vi "PPSU DC On.vi"(8 "Error in":errorcluster, 11 "Device information":string[](array[string])) -> (0 "Error out":errorcluster, 3 "Device information out":string[](array[string]))   [LabVIEW 2022 SP3]
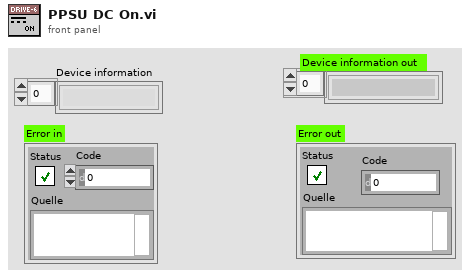
[diagram p1: front panel]
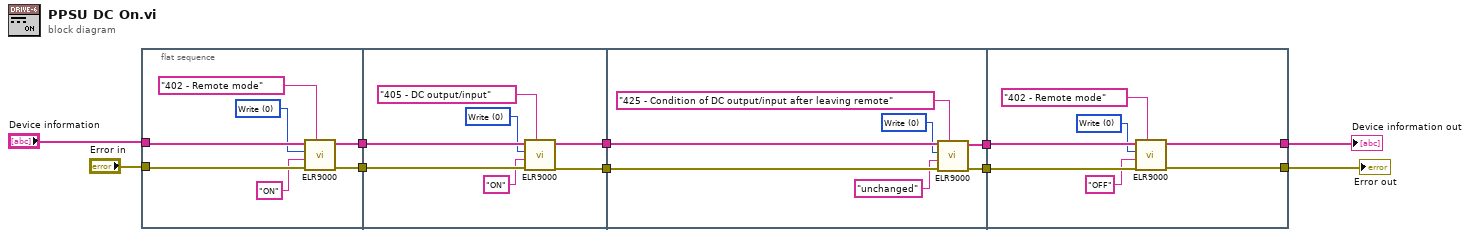
[diagram p0: block diagram]
diagram:
  n1 = flat-sequence {
    tunnel: "Error in" -> [w17]
    tunnel: "Device information" -> [w16]
    tunnel: [w12] -> w10
    tunnel: [w11] -> w9
    tunnel: w10 -> [w24]
    tunnel: w9 -> [w23]
    tunnel: [w19] -> w8
    tunnel: [w18] -> w7
    tunnel: w8 -> [w31]
    tunnel: w7 -> [w30]
    tunnel: [w26] -> w6
    tunnel: [w25] -> w5
    tunnel: w6 -> [w38]
    tunnel: w5 -> [w37]
    tunnel: [w33] -> w2
    tunnel: [w32] -> w1
    frame #0 {
      w14 = u8 0 items=["Write", "Read"] ("Access")
      n2 = call <vilib>:"ELR9000.vi"("Command list"="402 - Remote mode", "Error in"=w17, "Value"="ON", "Access"=w14, "Device information in"=w16) -> ("Error out"=w11:errorcluster, "Device information out"=w12:string[])  [unwired: 1 in, 2 out]
    }
    frame #1 {
      w21 = u8 0 items=["Write", "Read"] ("Access")
      n3 = call <vilib>:"ELR9000.vi"("Command list"="405 - DC output/input", "Error in"=w23, "Value"="ON", "Access"=w21, "Device information in"=w24) -> ("Error out"=w19:errorcluster, "Device information out"=w18:string[])  [unwired: 1 in, 2 out]
    }
    frame #2 {
      w29 = u8 0 items=["Write", "Read"] ("Access")
      n4 = call <vilib>:"ELR9000.vi"("Command list"="425 - Condition of DC output/input after leaving remote", "Error in"=w31, "Value"="unchanged", "Access"=w29, "Device information in"=w30) -> ("Error out"=w26:errorcluster, "Device information out"=w25:string[])  [unwired: 1 in, 2 out]
    }
    frame #3 {
      w35 = u8 0 items=["Write", "Read"] ("Access")
      n5 = call <vilib>:"ELR9000.vi"("Command list"="402 - Remote mode", "Error in"=w38, "Value"="OFF", "Access"=w35, "Device information in"=w37) -> ("Error out"=w32:errorcluster, "Device information out"=w33:string[])  [unwired: 1 in, 2 out]
    }
  }
  "Device information out" <- w2
  "Error out" <- w1
